vi "Read.vi"(6 "Append Index":i32, 8 "error in":errorcluster, 11 "ITX":refnum<class "Data.ITX.lvclass">) -> (0 "error out":errorcluster, 1 "Notes":string, 2 "Data (Dictionary)":T1[](array[typedef]), 3 "ITX out":refnum<class "Data.ITX.lvclass">, 5 "Path out":path)   [LabVIEW 2019, in "Data.ITX.lvclass"]
uses:
  Data.ITX.lvclass
  Data/Data.lvclass
  Data/Typedefs/Dictionary--cluster.ctl
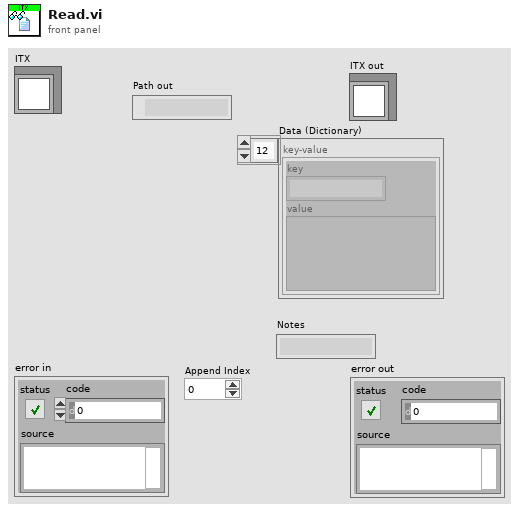
[diagram p1: front panel]
types:
  T1 = typedef "Data.lvclass/Dictionary--cluster.ctl" = cluster{"key":string, "value":variant}
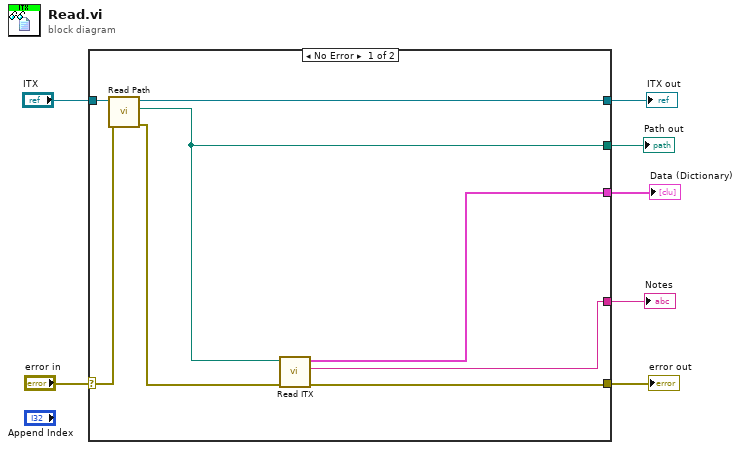
[diagram p0: block diagram]
diagram:
  n1 = case shown="No Error" "error in" {
    selector: "error in" -> [w11 w17]
    tunnel: "ITX" -> [w15 w16]
    tunnel: [w14 w16] -> w6
    tunnel: [w12 w17] -> w5
    tunnel: [w10 _] -> w3
    tunnel: [w8 _] -> w2
    tunnel: [w9 _] -> w1
    frame No Error {
      n2 = call "Read Path.vi"("error in (no error)"=w11, "Data Save"=w15) -> ("error out"=w13:errorcluster, "Path"=w10:path, "Data Save out"=w14:refnum<class "Data.ITX.lvclass">)  [unwired: 7 in]
      n3 = call "Read ITX.vi"("error in (no error)"=w13, "Path"=w10) -> ("error out"=w12:errorcluster, "Notes"=w9:string, "Data (Dictionary)"=w8:T1[])  [unwired: 6 in, 1 out]
    }
    frame Error {
    }
  }
  "error out" <- w5
  "ITX out" <- w6
  "Data (Dictionary)" <- w2
  "Path out" <- w3
  "Notes" <- w1
